vi "I2C_Detect.vi"(5 "Bus":i32=1, 6 "error in":errorcluster) -> (0 "error out":errorcluster, 4 "I2C Devices":u8[](array[numeric]) format="%.0x")   [LabVIEW 2014, in "Raspberry Pi Compatible Compiler for LabVIEW.lvlib" / "GPIO.lvlib"]
doc: "Scans for I2C devices on the specified bus.\n\nThis VI uses the same technique as the i2cdetect tool, consult the documentation for the known issues."
uses:
  GPIO.lvlib
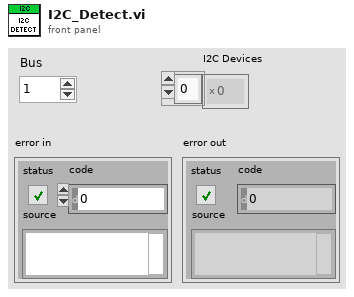
[diagram p1: front panel]
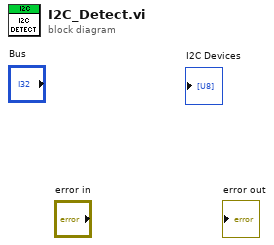
[diagram p0: block diagram]
diagram:
